vi "Query Meas name.vi"(6 "Channel":string="1", 7 "VISA resource name":refnum<visa-resource-name>="TCPIP0::A-N5225A-10057::inst0::INSTR", 8 "VNA Model":enum16{"E5071C", "N5230A(C)"}(ring)=enum."N5230A(C)") -> (0 "Parameter item":string[](array[string])=["Sdd21", "Sdd22", "Scd21", "Scd22"], 1 "Name list":string[](array[string])=["CH2_S11_7", "CH2_SDD22_8", "CH2_SCD21_9", "CH2_SCD22_10"], 3 "Dup VISA resource name":refnum<visa-resource-name>="TCPIP0::A-N5225A-10057::inst0::INSTR")   [LabVIEW 2011]
panel:
  out "read buffer":string="\"CH2_S11_7,Sdd21,CH2_SDD22_8,Sdd22,CH2_SCD21_9,Scd21,CH2_SCD22_10,Scd22\"\n"
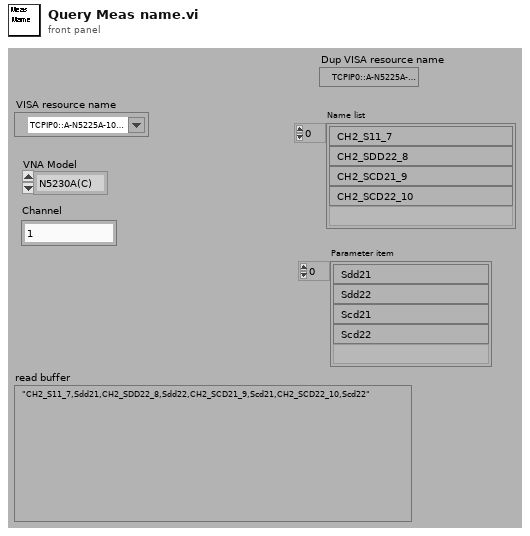
[diagram p1: front panel]
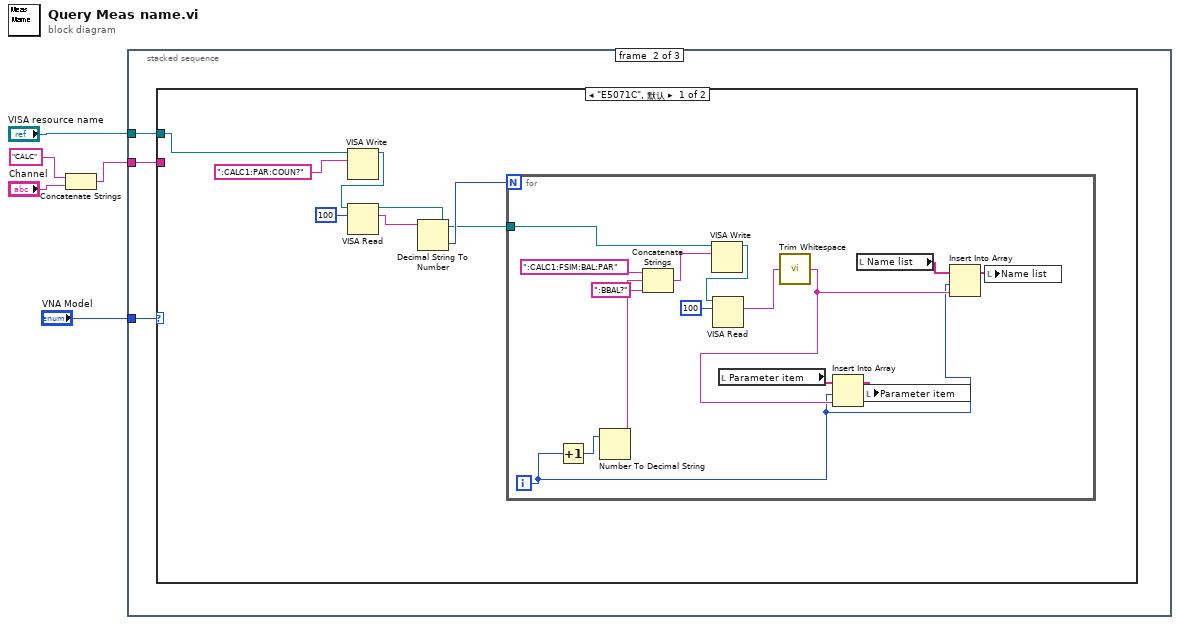
[diagram p0: block diagram]
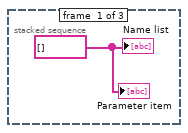
[diagram p2: hidden frame]
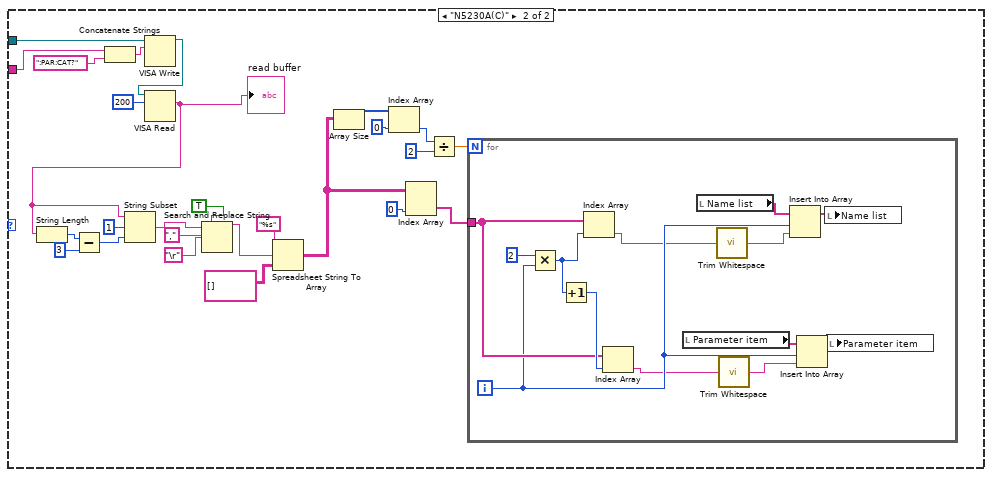
[diagram p3: hidden frame]
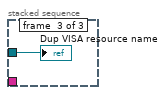
[diagram p4: hidden frame]
diagram:
  n1 = Concatenate Strings("CALC" ("字符串"), "Channel") -> (w1:string)
  n2 = stacked-sequence {
    tunnel: "VISA resource name" -> [_ w9 w71]
    tunnel: "VNA Model" -> [_ w8 _]
    tunnel: w1 -> [_ w7 _]
    frame #0 {
      w6 = string[] [] ("Name list")
      "Name list" <- w6
      "Parameter item" <- w6
    }
    frame #1 {
      n3 = case shown="\"E5071C\", 默认" w8 {
        tunnel: w9 -> [w14 w38]
        tunnel: w7 -> [_ w34]
        frame "E5071C", Default {
          n4 = VISA Write(VISA resource name=w14, write buffer=":CALC1:PAR:COUN?") -> (VISA resource name out=w13:refnum<visa-resource-name>)  [unwired: 1 in, 2 out]
          n5 = VISA Read(VISA resource name=w13, byte count=u32 100) -> (VISA resource name out=w10:refnum<visa-resource-name>, read buffer=w12:string)  [unwired: 1 in, 2 out]
          n6 = Decimal String To Number(string=w12) -> (number=w11:i32)  [unwired: 2 in, 1 out]
          n7 = for {
            N: w11 -> [_]
            tunnel: w10 -> [w31]
            i -> [w17]
            n8 = Increment(x=w17) -> (x+1=w29:i32)
            n9 = Number To Decimal String(number=w29) -> (decimal integer string=w28:string)  [unwired: 1 in]
            n10 = Concatenate Strings(":CALC1:FSIM:BAL:PAR" ("string"), w28, ":BBAL?" ("string")) -> (w30:string)
            n11 = VISA Write(VISA resource name=w31, write buffer=w30) -> (VISA resource name out=w25:refnum<visa-resource-name>)  [unwired: 1 in, 2 out]
            n12 = VISA Read(VISA resource name=w25, byte count=u32 100) -> (read buffer=w21:string)  [unwired: 1 in, 3 out]
            n13 = local read "Parameter item"() -> (w23:string[])
            n14 = call <vilib>:"Trim Whitespace.vi"("string"=w21) -> ("trimmed string"=w18:string)  [unwired: 1 in]
            n15 = Insert Into Array(array=w23, index=w17, new element=w18) -> (w22:string[])
            n16 = local read "Name list"() -> (w19:string[])
            n17 = local write "Parameter item"(w22) -> ()
            n18 = Insert Into Array(array=w19, index=w17, new element=w18) -> (w20:string[])
            n19 = local write "Name list"(w20) -> ()
          }
        }
        frame "N5230A(C)" {
          n20 = Concatenate Strings(w34, ":PAR:CAT?") -> (w32:string)
          n21 = VISA Write(VISA resource name=w38, write buffer=w32) -> (VISA resource name out=w36:refnum<visa-resource-name>)  [unwired: 1 in, 2 out]
          n22 = VISA Read(VISA resource name=w36, byte count=u32 200) -> (read buffer=w35:string)  [unwired: 1 in, 3 out]
          "read buffer" <- w35
          n23 = String Length(string=w35) -> (length=w50:i32)
          n24 = Subtract(x=w50, y=3) -> (x-y=w48:i32)
          n25 = String Subset(string=w35, offset (0)=1, length (rest)=w48) -> (substring=w47:string)
          n26 = Search and Replace String(replace all?=TRUE ("replace all? (F)"), input string=w47, search string=",", replace string="\r") -> (result string=w55:string)  [unwired: 4 in, 3 out]
          n27 = Spreadsheet String To Array(format string="%s", spreadsheet string=w55, array type (2D Dbl)=string[][] [] ("array 2")) -> (array=w44:string[][])  [unwired: 1 in]
          n28 = Array Size(array=w44) -> (size(s)=w46:i32[])
          n29 = Index Array(array=w46, index=0) -> (element=w41:i32)
          n30 = Index Array(array=w44, index (col)=0 ("disabled index (col)")) -> (element=w42:string[])  [unwired: 1 in]
          n31 = Divide(x=w41, y=2) -> (x/y=w39:dbl)
          n32 = for {
            N: w39 -> [_]
            tunnel: w42 -> [w65]
            i -> [w64]
            n33 = Multiply(x=2, y=w64) -> (x*y=w67:i32)
            n34 = Increment(x=w67) -> (x+1=w66:i32)
            n35 = Index Array(array=w65, index=w67) -> (element=w59:string)
            n36 = Index Array(array=w65, index=w66) -> (element=w61:string)
            n37 = local read "Parameter item"() -> (w63:string[])
            n38 = local read "Name list"() -> (w68:string[])
            n39 = call <vilib>:"Trim Whitespace.vi"("string"=w59) -> ("trimmed string"=w58:string)  [unwired: 1 in]
            n40 = call <vilib>:"Trim Whitespace.vi"("string"=w61) -> ("trimmed string"=w60:string)  [unwired: 1 in]
            n41 = Insert Into Array(array=w68, index=w64, new element=w58) -> (w69:string[])
            n42 = Insert Into Array(array=w63, index=w64, new element=w60) -> (w62:string[])
            n43 = local write "Name list"(w69) -> ()
            n44 = local write "Parameter item"(w62) -> ()
          }
        }
      }
    }
    frame #2 {
      "Dup VISA resource name" <- w71
    }
  }
